vi "GUI_map_image_parser.vi"(4 "zoom#":dbl=70.0, 5 "Image Src":T2, 6 "Ctl Refnum":refnum<vi>, 7 "Image Dst":T2, 8 "Image options":T1, 9 "size":cluster{"xhair size":dbl, "xhair size 2":dbl}={"xhair size"=20.0, "xhair size 2"=20.0} {"xhair size 2" min=0.0 max=0.0; "xhair size" min=0.0 max=0.0}, 10 "target y":dbl=0.001 caption="Y" min=0.0 max=2000.0, 11 "target x":dbl=0.001 caption="X" min=0.0 max=2000.0) -> (2 "ms timer out":u32, 3 "Img out":T2(plugin-control) caption="M1 Cam")   [LabVIEW 2013]
uses:
  <vilib>/vision/Image Controls.llb/IMAQ Image.ctl
  General/shared/Image GUI options.ctl
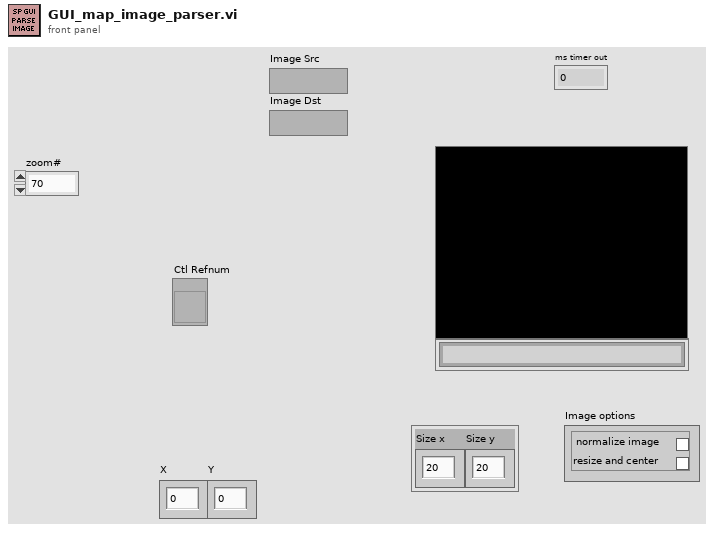
[diagram p1: front panel]
types:
  T1 = typedef "Image GUI options.ctl" = cluster{"normalize image":bool, "resize and center":bool}
  T2 = typedef "IMAQ Image.ctl" = refnum<image>
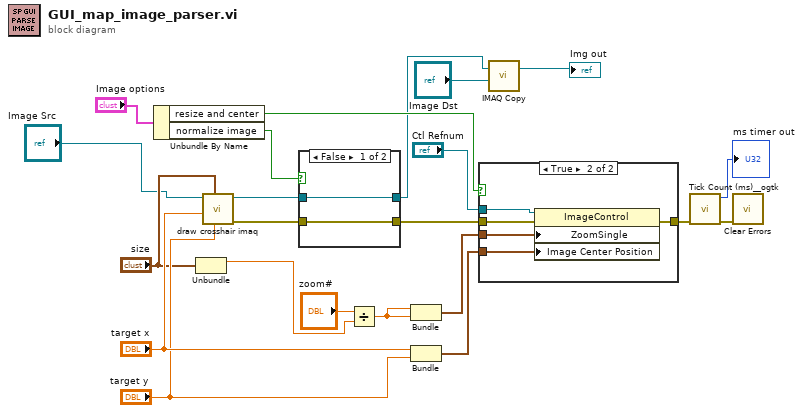
[diagram p0: block diagram]
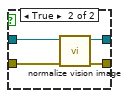
[diagram p2: hidden frame]
diagram:
  n1 = Unbundle By Name("Image options") -> ("resize and center"=w9:bool, "normalize image"=w4:bool)
  n2 = Unbundle("size") -> ("xhair size"=w6:dbl)  [unwired: 1 out]
  n3 = call "draw crosshair imaq.vi"("Target.Y"="target y", "size"="size", "Target.X"="target x", "image in"="Image Src") -> ("error out"=w7:errorcluster, "image out"=w22:T2)  [unwired: 6 in]
  n4 = case shown="False" w4 {
    tunnel: w22 -> [w24 w28]
    tunnel: [w24 w27] -> w1
    tunnel: [w23 w26] -> w14
    tunnel: w7 -> [w23 w25]
    frame False {
    }
    frame True {
      n5 = call "normalize vision image.vi"("error in (no error)"=w25, "Refnum in"=w28) -> ("error out"=w26:errorcluster, "Refnum out"=w27:T2)  [unwired: 7 in, 1 out]
    }
  }
  n6 = Divide(x="zoom#", y=w6) -> (x/y=w19:dbl)
  n7 = Bundle(w19, w19) -> (w21:cluster{dbl, dbl})  [unwired: 1 in]
  n8 = Bundle("target x"="target x", "target y"="target y") -> (w18:cluster{"target x":dbl, "target y":dbl})  [unwired: 1 in]
  n9 = case shown="True" w9 {
    tunnel: w21 -> [_ w34]
    tunnel: w18 -> [_ w33]
    tunnel: [w29 w32] -> w15
    tunnel: w14 -> [w29 w31]
    tunnel: "Ctl Refnum" -> [_ w30]
    frame False {
    }
    frame True {
      n10 = property on="Property Node" class="ImageControl"(reference=w30, error in=w31, "ZoomSingle"=w34, "Image Center Position"=w33) -> (error out=w32:errorcluster)  [unwired: 1 out]
    }
  }
  n11 = call "IMAQ Copy"("Image Dst"="Image Dst", "Image Src"=w1) -> ("Image Dst Out"=→"Img out":T2)  [unwired: 4 in, 1 out]
  n12 = call <userlib>:"Tick Count (ms)__ogtk.vi"("error in (no error)"=w15) -> ("error out"=w8:errorcluster, "millisecond timer value"=→"ms timer out":u32)  [unwired: 9 in]
  n13 = call <vilib>:"Clear Errors.vi"("error in (no error)"=w8) -> ()  [unwired: 6 in, 1 out]
